vi "path to stupid string.vi"(1 "Path":path) -> (0 "stupid string":string)   [LabVIEW 2016, in "connection creator.lvclass"]
uses:
  connection creator.lvclass
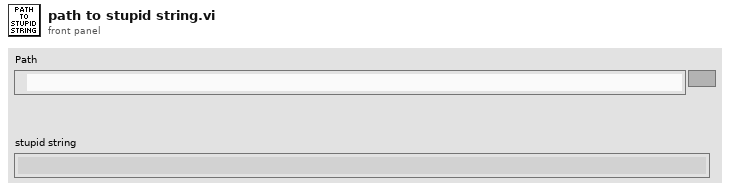
[diagram p1: front panel]
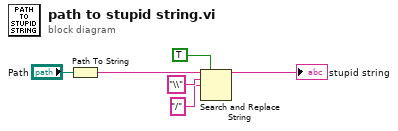
[diagram p0: block diagram]
diagram:
  n1 = Path To String(path="Path") -> (string=w5:string)
  n2 = Search and Replace String(replace all?=TRUE ("replace all? (F)"), input string=w5, search string="\\", replace string="/" ("replace string (\"\")")) -> (result string=→"stupid string":string)  [unwired: 4 in, 3 out]
